vi "Actor Core.vi"(8 "error in":errorcluster, 11 "Pressure in":refnum<class "Pressure.lvclass">) -> (0 "error out":errorcluster, 3 "Actor out":refnum<class "Actor.lvclass">)   [LabVIEW 2018, in "Pressure Actor.lvlib" / "Pressure.lvclass"]
doc: "(<B>Filename</B>: Actor Framework.lvlib:Actor.lvclass:Actor Core.vi)\n\nReceives messages to the actor, reacts to them, and initiates any error handling that may shut the actor down.\n\nDescendant classes may override this VI to append parallel tasks for the actor to complete while it handles messages. Overrides use the Call Parent Method node."
uses:
  Pressure.lvclass
  C:/Program Files/National Instruments/LabVIEW 2018/vi.lib/MGI/Panel Manager/Panel Actor/Panel Actor/Panel Actor.lvclass
  C:/Program Files/National Instruments/LabVIEW 2018/vi.lib/ActorFramework/Actor/Actor.lvclass
  <vilib>/ActorFramework/Actor/Actor.lvclass
  Pressure.lvclass/Pressure.ctl
  <vilib>/ActorFramework/Actor/Actor.lvclass/Actor.ctl
  <vilib>/ActorFramework/Message Enqueuer/Message Enqueuer.lvclass/Message Enqueuer.ctl
  <vilib>/ActorFramework/Message Enqueuer/Init from Existing Queue.vi
  <vilib>/ActorFramework/Message Enqueuer/Enqueue.vi
  Pressure Messages/Read Pressure Msg/Read Pressure Msg.lvclass
  C:/Program Files/National Instruments/LabVIEW 2018/vi.lib/ActorFramework/Message/Message.lvclass
  <vilib>/ActorFramework/Message Priority Queue/Priority Enqueue.vi
  <vilib>/ActorFramework/Message Enqueuer/Message Enqueuer.lvclass
  <vilib>/MGI/Panel Manager/Panel Actor/Panel Actor/Panel Actor.lvclass
  ADM/Main.lvlib
panel:
  out "Pressure":dbl format="%#_3g"
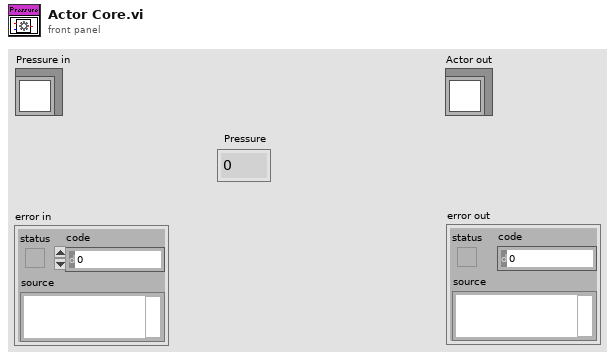
[diagram p1: front panel]
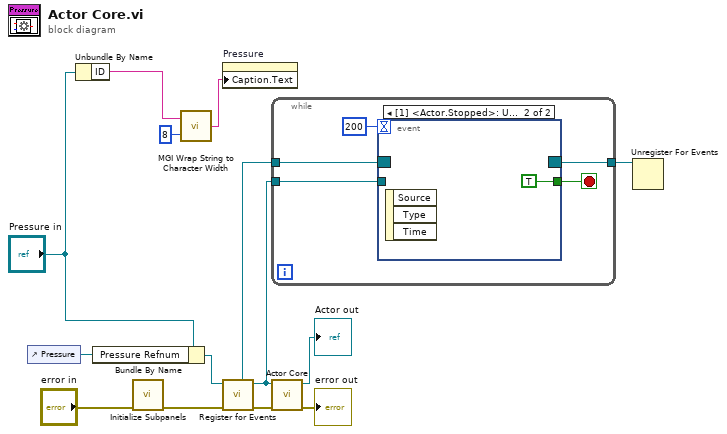
[diagram p0: block diagram]
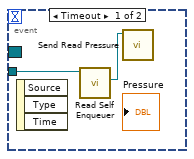
[diagram p2: hidden frame]
diagram:
  n1 = control-ref of="Pressure"() -> (w9:refnum<vi>)
  n2 = Unbundle By Name("Pressure in") -> ("ID"=w3:string)
  n3 = Bundle By Name(cluster="Pressure in", "Pressure Refnum"=w9) -> (w5:refnum<class "Pressure.lvclass">)
  n4 = call "Initialize Subpanels.vi"("error in (no error)"="error in") -> ("error out"=w8:errorcluster)  [unwired: 10 in]
  n5 = call <userlib>:"MGI Wrap String to Character Width.vi"("Wrap length(Characters)"=8, "Unwrapped string"=w3) -> ("Wrapped String"=w1:string)
  n6 = property on="Pressure" class="DigNum (strict)"("Caption.Text"=w1) -> ()  [unwired: 2 in, 2 out]
  n7 = call <vilib>:"Register for Events.vi"("Error In"=w8, "Panel Actor in"=w5) -> ("Error Out"=w6:errorcluster, "Panel Actor out"=w4:refnum<class "Pressure.lvclass">, "Pnl Actor"=w7:refnum<event-registration>)  [unwired: 6 in, 1 out]
  n8 = while {
    tunnel: w7 -> [w19]
    tunnel: [w18] -> w12
    tunnel: w4 -> [w15]
    stop <- w17 stop-if-true
    n9 = event shown="[1] <Actor.Stopped>: User Event" {
      selector: w19 -> [_ _]
      dyn-events: [_ _] -> w18
      timeout: 200 -> [_ _]
      tunnel: [_ TRUE] -> w17
      tunnel: w15 -> [w21 _]
      event Timeout {
        n10 = event-data() -> ()  [unwired: 1 in, 3 out]
        n11 = call <vilib>:"Read Self Enqueuer.vi"("Actor"=w21) -> ("Self Enqueuer"=w20:refnum<class "Message Enqueuer.lvclass">)  [unwired: 10 in]
        n12 = call "Send Read Pressure.vi"("Message Enqueuer in"=w20) -> ()  [unwired: 9 in, 2 out]
      }
      event User Event {
        n13 = event-data() -> ()  [unwired: 1 in, 3 out]
      }
    }
  }
  n14 = call-parent "Actor Core.vi"("error in"=w6, "Panel Actor in"=w4) -> ("error out"=→"error out":errorcluster, "Actor out"=→"Actor out":refnum<class "Actor.lvclass">)  [unwired: 8 in]
  n15 = Unregister For Events(event registration refnum=w12) -> ()  [unwired: 1 in, 1 out]
